vi "pre-processamento.vi"() -> (0 "TimeStamp":dynamicdata(graph), 1 "Waveform Graph 3":dbl[](graph) caption="Potência Ativa C", 2 "Waveform Graph 2":dbl[](graph) caption="Potência Ativa B", 3 "Waveform Graph":dbl[](graph) caption="Potência Ativa A")   [LabVIEW 2020]
uses:
  <vilib>/numeric/Random Number (Range) DBL.vi
panel:
  out "fator de potência 3":dbl
  out "Potencia \nativa C":string[][](table)
  out "Tensão e Corrent C":string[][](table)
  out "fator de potência 2":dbl
  out "Potencia \nativa B":string[][](table)
  out "Tensão e Corrent B":string[][](table)
  out "fator de potência":dbl
  out "Potencia \nativa":string[][](table)
  out "Tensão e Corrent A":string[][](table)
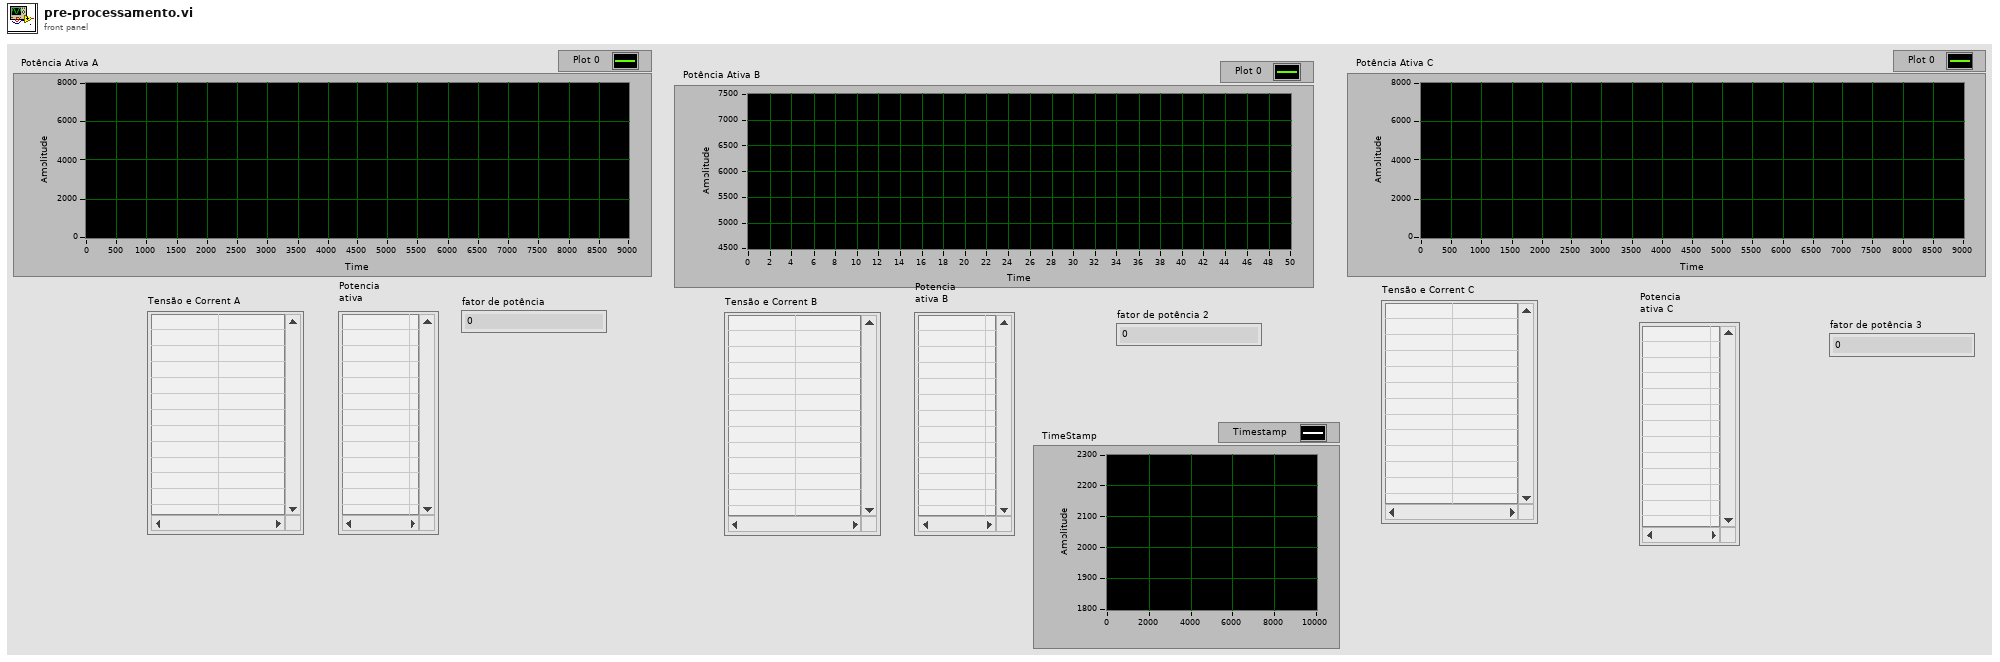
[diagram p1: front panel]
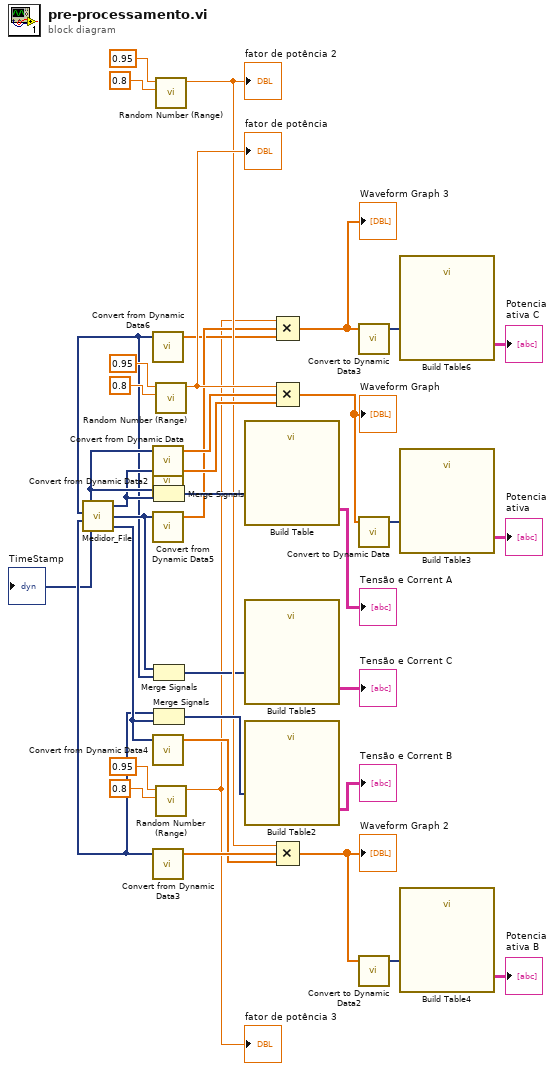
[diagram p0: block diagram]
diagram:
  n1 = call "Medidor_File.vi"() -> ("Corrente Fase C"=w15:dynamicdata, "Corrente Fase B"=w3:dynamicdata, "Corrente Fase A"=w30:dynamicdata, "TimeStamp"=→"TimeStamp":dynamicdata, "Tensão Fase C"=w14:dynamicdata, "Tensão Fase B"=w2:dynamicdata, "Tensão Fase A"=w31:dynamicdata)
  n2 = call "Convert from Dynamic Data6"("Dynamic Data Type"=w2) -> ("Array"=w12:dbl[])  [unwired: 3 in]
  n3 = call "Convert from Dynamic Data"("Dynamic Data Type"=w31) -> ("Array"=w37:dbl[])  [unwired: 3 in]
  n4 = call "Convert from Dynamic Data2"("Dynamic Data Type"=w30) -> ("Array"=w36:dbl[])  [unwired: 3 in]
  n5 = call "Convert from Dynamic Data5"("Dynamic Data Type"=w3) -> ("Array"=w13:dbl[])  [unwired: 3 in]
  n6 = call "Convert from Dynamic Data4"("Dynamic Data Type"=w15) -> ("Array"=w24:dbl[])  [unwired: 3 in]
  n7 = call "Convert from Dynamic Data3"("Dynamic Data Type"=w14) -> ("Array"=w25:dbl[])  [unwired: 3 in]
  n8 = Merge Signals(w31, w30) -> (w29:dynamicdata)
  n9 = Merge Signals(w3, w2) -> (w7:dynamicdata)
  n10 = Merge Signals(w14, w15) -> (w19:dynamicdata)
  n11 = call-poly <vilib>:"Random Number (Range).vi"("lower bound (0)"=0.8, "upper bound (100)"=0.95) -> ("number"=w16:dbl)  [unwired: 9 in]
  "fator de potência 2" <- w16
  n12 = call-poly <vilib>:"Random Number (Range).vi"("lower bound (0)"=0.8, "upper bound (100)"=0.95) -> ("number"=w26:dbl)  [unwired: 9 in]
  "fator de potência" <- w26
  n13 = call-poly <vilib>:"Random Number (Range).vi"("lower bound (0)"=0.8, "upper bound (100)"=0.95) -> ("number"=w4:dbl)  [unwired: 9 in]
  "fator de potência 3" <- w4
  n14 = call "Build Table"("Signals"=w29) -> ("Table"=→"Tensão e Corrent A":string[][])  [unwired: 4 in, 6 out]
  n15 = call "Build Table5"("Signals"=w7) -> ("Table"=→"Tensão e Corrent C":string[][])  [unwired: 4 in, 6 out]
  n16 = call "Build Table2"("Signals"=w19) -> ("Table"=→"Tensão e Corrent B":string[][])  [unwired: 4 in, 6 out]
  n17 = Compound Arithmetic op=MULTIPLY(w4, w13, w12) -> (w9:dbl[])
  "Waveform Graph 3" <- w9
  n18 = Compound Arithmetic op=MULTIPLY(w26, w37, w36) -> (w33:dbl[])
  "Waveform Graph" <- w33
  n19 = Compound Arithmetic op=MULTIPLY(w16, w25, w24) -> (w21:dbl[])
  "Waveform Graph 2" <- w21
  n20 = call "Convert to Dynamic Data3"("Array"=w9) -> ("Dynamic Data Type"=w8:dynamicdata)  [unwired: 3 in]
  n21 = call "Convert to Dynamic Data"("Array"=w33) -> ("Dynamic Data Type"=w32:dynamicdata)  [unwired: 3 in]
  n22 = call "Convert to Dynamic Data2"("Array"=w21) -> ("Dynamic Data Type"=w20:dynamicdata)  [unwired: 3 in]
  n23 = call "Build Table6"("Signals"=w8) -> ("Table"=→"Potencia \nativa C":string[][])  [unwired: 4 in, 6 out]
  n24 = call "Build Table3"("Signals"=w32) -> ("Table"=→"Potencia \nativa":string[][])  [unwired: 4 in, 6 out]
  n25 = call "Build Table4"("Signals"=w20) -> ("Table"=→"Potencia \nativa B":string[][])  [unwired: 4 in, 6 out]
